vi "位置模式测试.vi"() -> ()   [LabVIEW 2013]
panel:
  out "位置":dbl=10000.0
  in  "Change Velocity":dbl=1.0
  in  "Distance":dbl
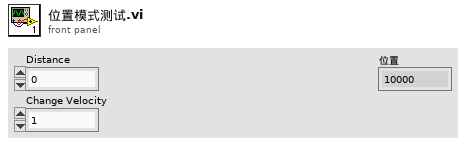
[diagram p1: front panel]
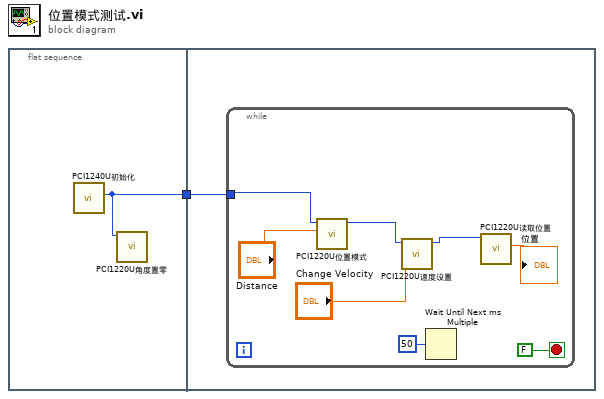
[diagram p0: block diagram]
diagram:
  n1 = flat-sequence {
    tunnel: [w2] -> w1
    tunnel: w1 -> [w3]
    frame #0 {
      n2 = call "PCI1240U初始化.vi"() -> ("X电机"=w2:u32)  [unwired: 6 in, 5 out]
      n3 = call "PCI1220U角度置零.vi"("AxisHandle IN"=w2) -> ()  [unwired: 10 in, 1 out]
    }
    frame #1 {
      n4 = while {
        tunnel: w3 -> [w8]
        stop <- FALSE stop-if-true
        n5 = call "PCI1220U位置模式.vi"("Distance"="Distance", "AxisHandle IN"=w8) -> ("AxisHandle OUT"=w7:u32)  [unwired: 8 in, 1 out]
        n6 = call "PCI1220U速度设置.vi"("Change Velocity"="Change Velocity", "AxisHandle IN"=w7) -> ("AxisHandle OUT"=w5:u32)  [unwired: 9 in]
        n7 = Wait Until Next ms Multiple(millisecond multiple=u32 50 ("毫秒倍数")) -> ()  [unwired: 1 out]
        n8 = call "PCI1220U读取位置.vi"("AxisHandle IN"=w5) -> ("位置"=→"位置":dbl)  [unwired: 9 in, 1 out]
      }
    }
  }
